vi "ke37xx Error Query.vi"(0 "VISA resource name":refnum<visa-resource-name>, 11 "error in (no error)":errorcluster) -> (4 "VISA resource name out":refnum<visa-resource-name>, 8 "Error":i32, 10 "Error Message":string, 15 "error out":errorcluster)   [LabVIEW 2019, in "Keithley 3700 Series.lvlib"]
doc: "This VI reads an error from the instrument. It expects to see errors in SCPI format (#,\"error message\"). If an error query is not supported, it returns a warning."
uses:
  Keithley 3700 Series.lvlib
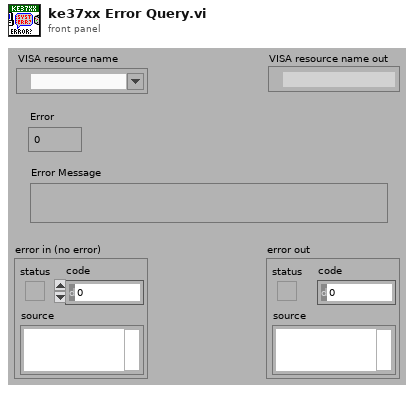
[diagram p1: front panel]
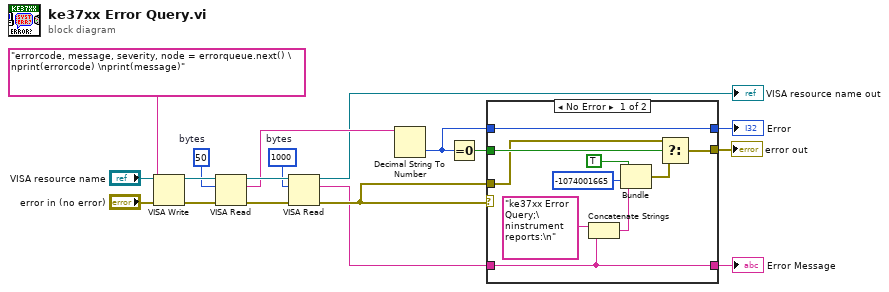
[diagram p0: block diagram]
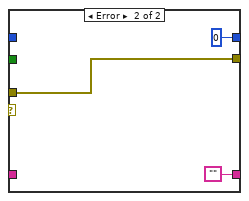
[diagram p2: hidden frame]
diagram:
  w2 = u32 1000  # bytes
  w3 = u32 50  # bytes
  n1 = VISA Write(VISA resource name="VISA resource name", write buffer="errorcode, message, severity, node = errorqueue.next() \nprint(errorcode) \nprint(message)", error in (no error)="error in (no error)") -> (VISA resource name out=w16:refnum<visa-resource-name>, error out=w10:errorcluster)  [unwired: 1 out]
  n2 = VISA Read(VISA resource name=w16, byte count=w3, error in (no error)=w10) -> (VISA resource name out=w17:refnum<visa-resource-name>, read buffer=w12:string, error out=w1:errorcluster)  [unwired: 1 out]
  n3 = VISA Read(VISA resource name=w17, byte count=w2, error in (no error)=w1) -> (VISA resource name out=→"VISA resource name out":refnum<visa-resource-name>, read buffer=w4:string, error out=w18:errorcluster)  [unwired: 1 out]
  n4 = Decimal String To Number(string=w12) -> (number=w9:i32)  [unwired: 3 out]
  n5 = Equal To 0?(x=w9) -> (x = 0?=w11:bool)
  n6 = case shown="No Error" w18 {
    tunnel: w4 -> [w26 _]
    tunnel: [w20 w29] -> w6
    tunnel: [w26 "" ("Empty String Constant")] -> w14
    tunnel: [w24 0] -> w13
    tunnel: w9 -> [w24 _]
    tunnel: w11 -> [w23 _]
    tunnel: w18 -> [w21 w29]
    frame No Error {
      n7 = Concatenate Strings("ke37xx Error Query;\ninstrument reports:\n", w26) -> (w25:string)
      n8 = Bundle(TRUE, -1074001665, w25) -> (w22:errorcluster)  [unwired: 1 out]
      n9 = Select(t=w21, s=w23, f=w22) -> (s? t:f=w20:errorcluster)
    }
    frame Error {
    }
  }
  "Error Message" <- w14
  "Error" <- w13
  "error out" <- w6
